vi "Generate Arguments.vi"(7 "subsystem?":bool, 8 "error in (no error)":errorcluster, 9 "command":string, 11 "client in":refnum<class "Generic Client.lvclass">) -> (0 "error out":errorcluster, 2 "arguments":string[](array[string]), 3 "client out":refnum<class "Generic Client.lvclass">, 5 "environment variables":cluster{"name":string, "value":string}[](array[cluster]))   [LabVIEW 2020, in "NI_SSH.lvlib" / "Generic Client.lvclass"]
uses:
  <vilib>/net/SSH/Client/Generic/Generic Client.lvclass
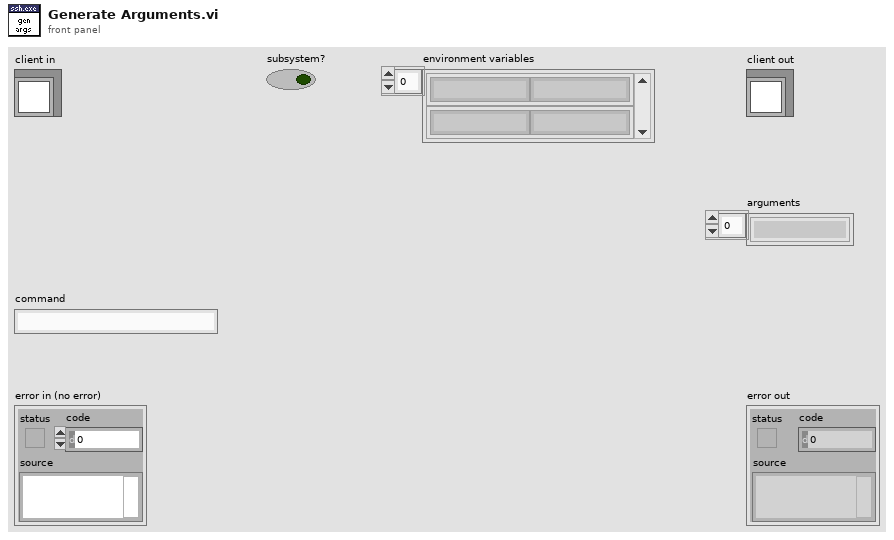
[diagram p1: front panel]
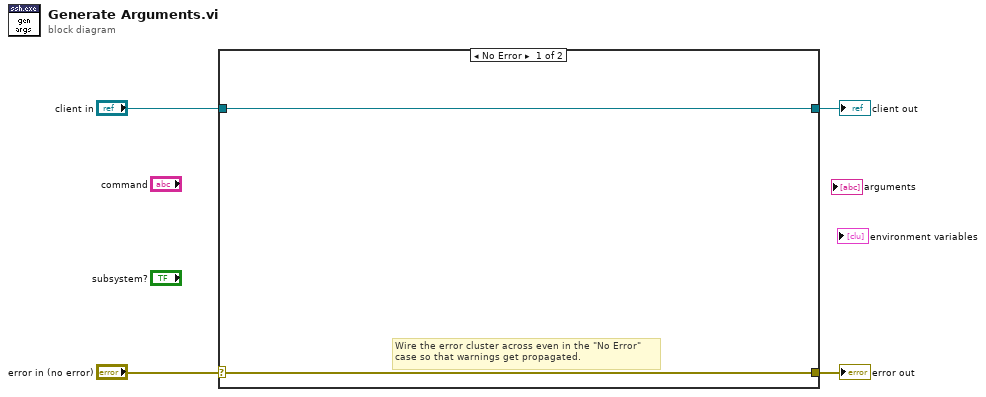
[diagram p0: block diagram]
diagram:
  n1 = case shown="No Error" "error in (no error)" {
    selector: "error in (no error)" -> [w5 w8]
    tunnel: [w5 w8] -> w3
    tunnel: [w6 w7] -> w1
    tunnel: "client in" -> [w6 w7]
    frame No Error {
      # "Wire the error cluster across even in the \"No Error\"\ncase so that warnings get propagated."
    }
    frame Error {
    }
  }
  "error out" <- w3
  "client out" <- w1
